vi "PSTR-Show Fit Summary.vi"(0 "Data":T1, 5 "XYGraph":refnum<vi>, 9 "Freq index":i32) -> ()   [LabVIEW 2020]
uses:
  Typedefs/PSTR-Data.ctl
  Typedefs/PSTR-Model Fit.ctl
  Typedefs/PSTR-Fit Parameters.ctl
panel:
  # "NF x NL x 2 x Npts"
  # "NF x NL x Npts"
  # "NF x NL"
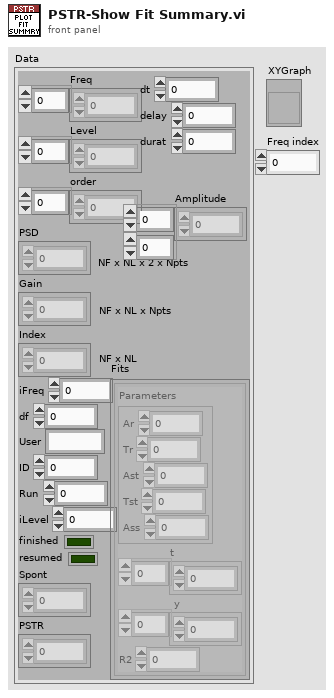
[diagram p1: front panel]
types:
  T1 = typedef "PSTR-Data.ctl" = cluster{"Freq":dbl[], "Level":dbl[], "order":i32[], "PSD":dbl[][][][], "Gain":dbl[][][], "Index":dbl[][], "iFreq":i32, "df":dbl, "User":string, "ID":i32, "Run":i32, "iLevel":i32, "finished":bool, "resumed":bool, "Spont":dbl[][], "PSTR":dbl[][][], "dt":dbl, "delay":dbl, "durat":dbl, "Fits":T2[][], "Amplitude":dbl[][]}
  T2 = typedef "PSTR-Model Fit.ctl" = cluster{"Parameters":T3, "t":dbl[], "y":dbl[], "R2":dbl}
  T3 = typedef "PSTR-Fit Parameters.ctl" = cluster{"Ar":dbl, "Tr":dbl, "Ast":dbl, "Tst":dbl, "Ass":dbl}
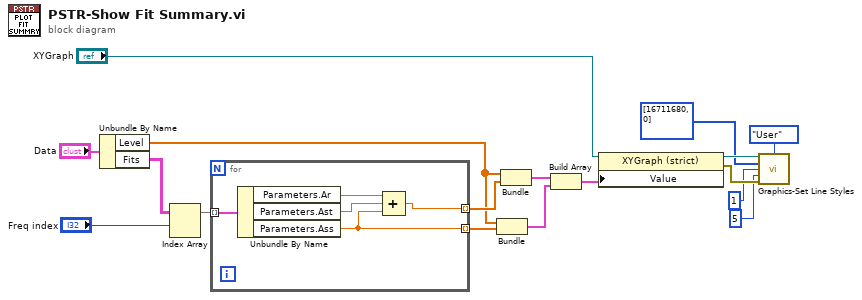
[diagram p0: block diagram]
diagram:
  n1 = Unbundle By Name("Data") -> ("Level"=w5:dbl[], "Fits"=w16:T2[][])
  n2 = Index Array(array=w16, index (row)="Freq index") -> (element=w7:T2[])  [unwired: 1 in]
  n3 = for {
    tunnel: w7 -> [w22] mode=indexing
    tunnel: [w19] -> w8 mode=indexing
    tunnel: [w18] -> w4 mode=indexing
    n4 = Unbundle By Name(w22) -> ("Parameters.Ar"=w21:dbl, "Parameters.Ast"=w20:dbl, "Parameters.Ass"=w18:dbl)
    n5 = Compound Arithmetic op=ADD(w21, w20, w18) -> (w19:dbl)
  }
  n6 = Bundle("Level"=w5, w4) -> (w2:cluster{"Level":dbl[], dbl[]})  [unwired: 1 in]
  n7 = Bundle("Level"=w5, w8) -> (w15:cluster{"Level":dbl[], dbl[]})  [unwired: 1 in]
  n8 = Build Array(w15, w2) -> (w3:cluster{"Level":dbl[], dbl[]}[])
  n9 = property class="XYGraph (strict)"(reference="XYGraph", "Value"=w3) -> (reference out=w13:refnum<vi>, error out=w12:errorcluster)  [unwired: 1 in]
  n10 = call "Graphics-Set Line Styles.vi"("XY Graph"=w13, "Map"=enum16{"User", "Prism", "Kelly", "Dark2"}."User", "Colors"=u32[] [16711680, 0], "Plot.Line Width"=u8 1, "Plot.Point Style"=u8 5, "error in (no error)"=w12) -> ()  [unwired: 8 in, 2 out]
